vi "set control settings calb.vi"(8 "error in (no error)":errorcluster, 9 "calibration":cluster{"A":dbl, "MicrostepMode":u32}, 10 "control_settings_calb":T1, 11 "id":i32) -> (0 "error out":errorcluster, 3 "function return":i32)   [LabVIEW 2012, in "libximc.lvlib"]
doc: "result_t XIMC_API set_control_settings_calb (device_t id, const control_settings_calb_t* control_settings_calb, const calibration_t* calibration);"
uses:
  libximc.lvlib
  libximc.dll
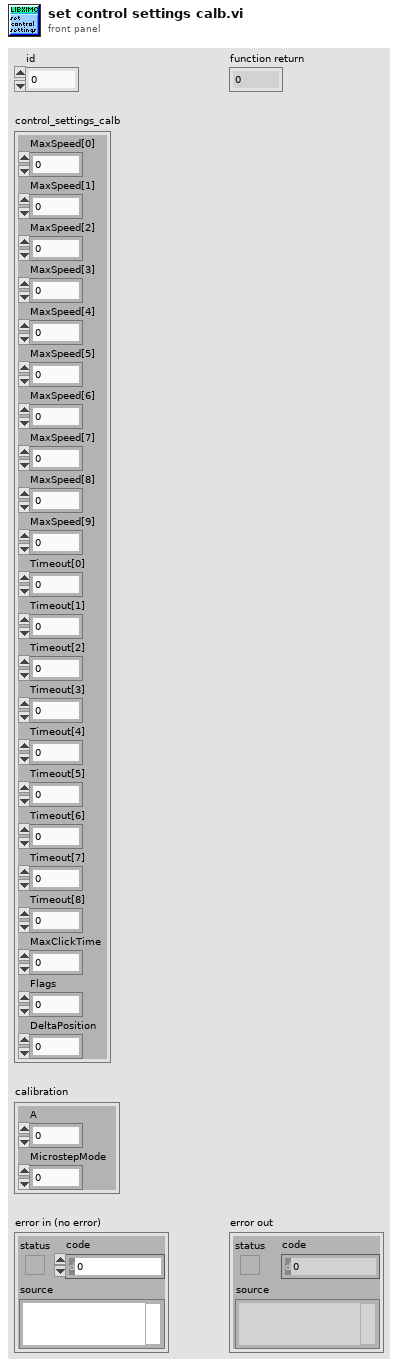
[diagram p1: front panel]
types:
  T1 = cluster{"MaxSpeed[0]":sgl, "MaxSpeed[1]":sgl, "MaxSpeed[2]":sgl, "MaxSpeed[3]":sgl, "MaxSpeed[4]":sgl, "MaxSpeed[5]":sgl, "MaxSpeed[6]":sgl, "MaxSpeed[7]":sgl, "MaxSpeed[8]":sgl, "MaxSpeed[9]":sgl, "Timeout[0]":u32, "Timeout[1]":u32, "Timeout[2]":u32, "Timeout[3]":u32, "Timeout[4]":u32, "Timeout[5]":u32, "Timeout[6]":u32, "Timeout[7]":u32, "Timeout[8]":u32, "MaxClickTime":u32, "Flags":u32, "DeltaPosition":sgl}
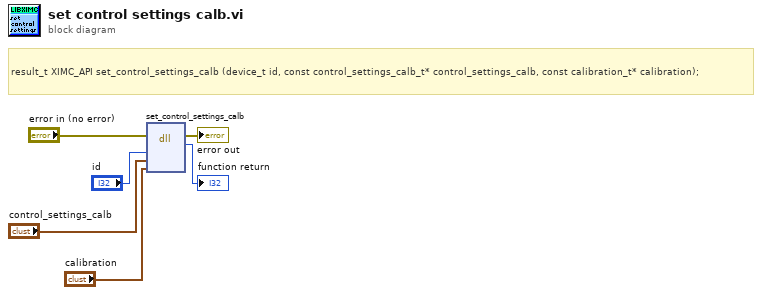
[diagram p0: block diagram]
diagram:
  # "result_t XIMC_API set_control_settings_calb (device_t id, const control_settings_calb_t* control_settings_calb, const calibration_t* calibration);"
  n1 = dll-call lib="C:/Users/Stepan/Downloads/labview_2.9.11_testgen_thread/libximc.*" fn="set_control_settings_calb"(error in="error in (no error)", "id"="id", "control_settings_calb"="control_settings_calb", "calibration"="calibration") -> (error out=→"error out":errorcluster, →"function return":i32)  [unwired: 5 in, 1 out]
